vi "Apply Transforms.vi"(8 "error in":errorcluster, 10 "Matrix":T1, 11 "Element in":refnum<class "Element.lvclass">) -> (0 "error out":errorcluster, 3 "Element out":refnum<class "Element.lvclass">)   [LabVIEW 2019, in "Element.lvclass"]
uses:
  Element.lvclass
  <vilib>/Analysis/NI_AALBase.lvlib
  <vilib>/Analysis/baseanly.llb/Real A x B.vi
  <vilib>/Analysis/Matrix/NI_Matrix.lvlib
  <vilib>/Analysis/Matrix/Numeric/Conversions/Array To Matrix - RA.vi
  <vilib>/Analysis/Matrix/Numeric/Conversions/Matrix To Array - RM.vi
  <vilib>/Analysis/Matrix/Datatypes/RealMatrix.ctl
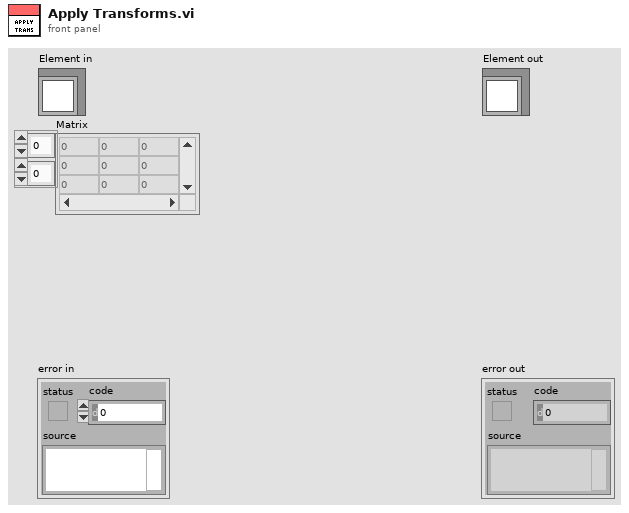
[diagram p1: front panel]
types:
  T1 = typedef "NI_Matrix.lvlib/RealMatrix.ctl" = dbl[][]
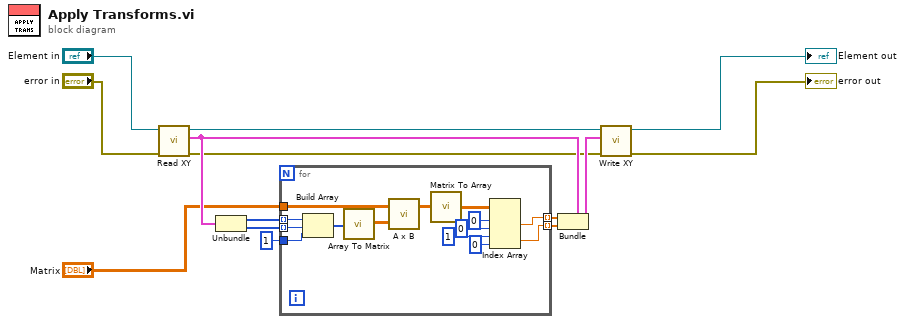
[diagram p0: block diagram]
diagram:
  n1 = call-dynamic "Read XY.vi"("error in (no error)"="error in", "Element in"="Element in") -> ("error out"=w3:errorcluster, "XY"=w13:cluster{"X":i32[], "Y":i32[]}, "Element out"=w14:refnum<class "Element.lvclass">)  [unwired: 7 in]
  n2 = Unbundle(w13) -> ("X"=w11:i32[], "Y"=w10:i32[])
  n3 = for {
    tunnel: w11 -> [w28] mode=indexing
    tunnel: w10 -> [w27] mode=indexing
    tunnel: 1 -> [w26]
    tunnel: "Matrix" -> [w24]
    tunnel: [w16] -> w8 mode=indexing
    tunnel: [w15] -> w7 mode=indexing
    n4 = Build Array(w28, w27, w26) -> (w25:i32[])
    n5 = call-poly <vilib>:"Array To Matrix.vi"("Real 1D Array"=w25) -> ("Real Matrix (Column Vector)"=w23:T1)
    n6 = call-poly <vilib>:"A x B.vi"("B"=w23, "A"=w24) -> ("A x B"=w22:T1)  [unwired: 1 out]
    n7 = call-poly <vilib>:"Matrix To Array.vi"("Real Matrix"=w22) -> ("Real 2D Array"=w21:dbl[][])
    n8 = Index Array(array=w21, index (row) #1=0 ("index (row)"), index (col) #1=0 ("disabled index (col)"), index (row) #2=1 ("index (row)"), index (col) #2=0 ("disabled index (col)")) -> (element #1=w16:dbl, element #2=w15:dbl)
  }
  n9 = Bundle(cluster=w13, "X"=w8, "Y"=w7) -> (w12:cluster{"X":i32[], "Y":i32[]})
  n10 = call-dynamic "Write XY.vi"("error in (no error)"=w3, "XY"=w12, "Element in"=w14) -> ("error out"=→"error out":errorcluster, "Element out"=→"Element out":refnum<class "Element.lvclass">)  [unwired: 7 in]
